vi "reasponse_body.vi"(7 "save_to_file":path, 8 "error in (no error)":errorcluster, 11 "Request in":refnum<class "Request.lvclass">) -> (0 "error out":errorcluster, 2 "string_value":string, 3 "Request in":refnum<class "Request.lvclass">)   [LabVIEW 2020, in "reqwest.lvlib" / "Request.lvclass"]
uses:
  Request/Request.lvclass
  Request/Request.lvclass/Request.ctl
  <userlib>/_OpenG.lib/file/file.llb/Valid Path - Traditional__ogtk.vi
  reqwest.lvlib
  <userlib>/_OpenG.lib/file/file.llb/openg_file.lvlib
  lv_reqwest_64.so
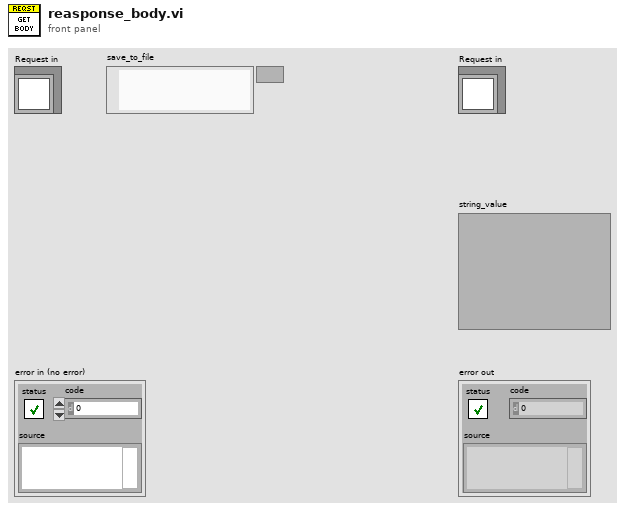
[diagram p1: front panel]
types:
  T1 = typedef "reqwest.lvlib/Request.lvclass/request_id_int.ctl" = u64
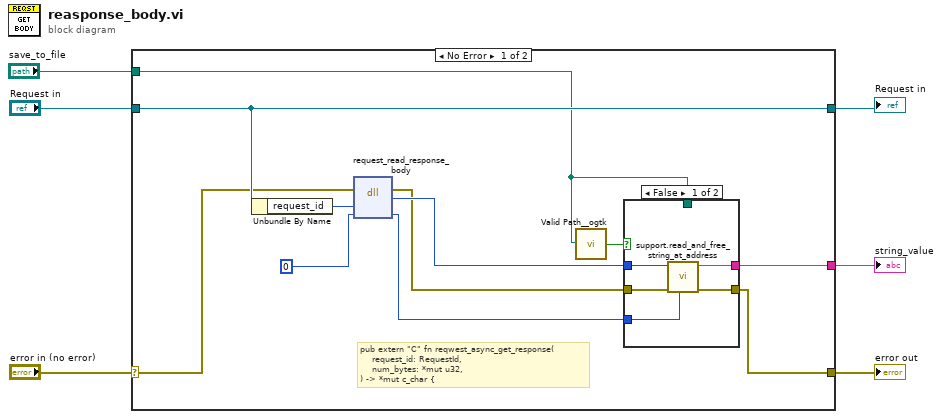
[diagram p0: block diagram]
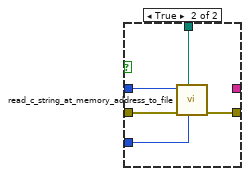
[diagram p2: hidden frame]
diagram:
  n1 = case shown="No Error" "error in (no error)" {
    selector: "error in (no error)" -> [w12 w28]
    tunnel: "Request in" -> [w13 w29]
    tunnel: [w14 _] -> w4
    tunnel: [w11 w28] -> w2
    tunnel: [w13 w29] -> w3
    tunnel: "save_to_file" -> [w7 _]
    frame No Error {
      # "pub extern \"C\" fn reqwest_async_get_response(\n    request_id: RequestId,\n    num_bytes: *mut u32,\n) -> *mut c_char {"
      n2 = Unbundle By Name(w13) -> ("request_id"=w15:T1)
      n3 = dll-call lib="home/jim-kring/Projects/reqwest-rs-labview/lv_src/lv_reqwest_*.*" fn="request_read_response_body"(error in=w12, "request_id"=w15, "num_bytes"=u32 0) -> (error out=w16:errorcluster, "string_ptr"=w17:u64, "num_bytes"=w9:u32)  [unwired: 3 in, 1 out]
      n4 = call-poly <userlib>:"Valid Path__ogtk.vi"("path"=w7) -> ("valid"=w8:bool)
      n5 = case shown="False" w8 {
        tunnel: w17 -> [w22 w25]
        tunnel: w16 -> [w21 w27]
        tunnel: [w20 _] -> w14
        tunnel: [w19 w26] -> w11
        tunnel: w9 -> [w18 w24]
        tunnel: w7 -> [_ w23]
        frame False {
          n6 = call "support.read_and_free_string_at_address.vi"("string_length"=w18, "error in (no error)"=w21, "string_ptr"=w22) -> ("error out"=w19:errorcluster, "string"=w20:string)  [unwired: 7 in]
        }
        frame True {
          n7 = call "read_c_string_at_memory_address_to_file.vi"("string_length"=w24, "File Path"=w23, "error in (no error)"=w27, "memory_address"=w25) -> ("error out"=w26:errorcluster)  [unwired: 6 in, 1 out]
        }
      }
    }
    frame Error {
    }
  }
  "error out" <- w2
  "string_value" <- w4
  "Request in" <- w3
